vi "add ch config.vi"(7 "range":string[](array[string]), 8 "CAl":T4, 9 "device chanel":T5 {"display" format="%b"}, 10 "value":string[](array[string]), 11 "Enum":T6=enum."CName") -> (2 "device chanel out":T5 {"display" format="%b"})   [LabVIEW 2011]
uses:
  singlechtype.ctl
  config table enum.ctl
  signal type.ctl
  gain.ctl
panel:
  in  "Enum 2":T1(ring)=enum."><（在范围外）"
  in  "Gain":T2
  in  "type":T3
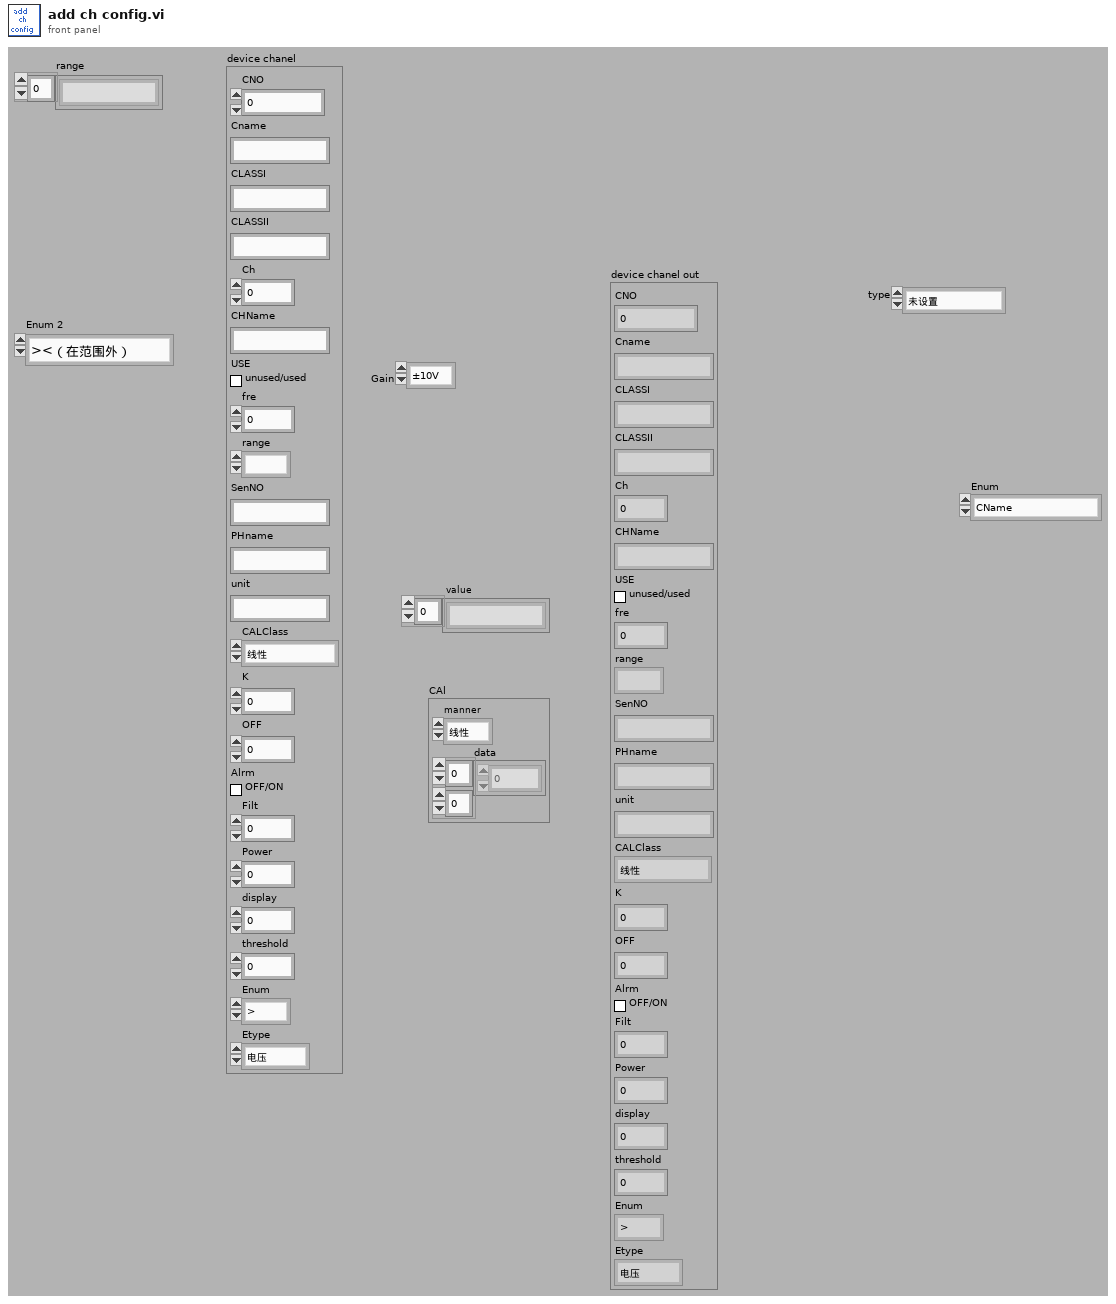
[diagram p1: front panel]
types:
  T1 = enum16{">", ">=", "<", "<=", "<>(在范围内）", "><（在范围外）"}
  T2 = typedef "gain.ctl" = enum16{"±10V", "±5V", "±2.5V", "±1V", "±500mV", "±100mV", "10V", "5V", "2.5V", "1V", "500mV", "100mV"}
  T3 = typedef "signal type.ctl" = enum16{"未设置", "volet", "current", "vibration", "electric charge ", "resistance "}
  T4 = cluster{"manner":enum16{"线性", "查表"}, "data":dbl[][]}
  T5 = typedef "singlechtype.ctl" = cluster{"CNO":u8, "Cname":string, "CLASSI":string, "CLASSII":string, "Ch":u8, "CHName":string, "USE":bool, "fre":dbl, "range":enum16{""}, "SenNO":string, "PHname":string, "unit":string, "CALClass":enum8{"线性", "查表", "公式"}, "K":dbl, "OFF":dbl, "Alrm":bool, "Filt":dbl, "Power":u8, "display":u8, "threshold ":dbl, "Enum":enum16{">", ">=", "<", "<=", "<>(在范围内）", "><（在范围外）"}, "Etype":enum16{"电压", "电流", "电阻", "热电偶K", "热电偶T"}}
  T6 = typedef "config table enum.ctl" = enum16{"CNO.", "CName", "CLASSI", "CLASSII", "ch", "Chname", "USE", "fre", "range", "senNO", "PHname", "unit", "CALclass", "K", "OFF", "Alrm", "filt", "Power", "display", "threshold", "compare", "Etype"}
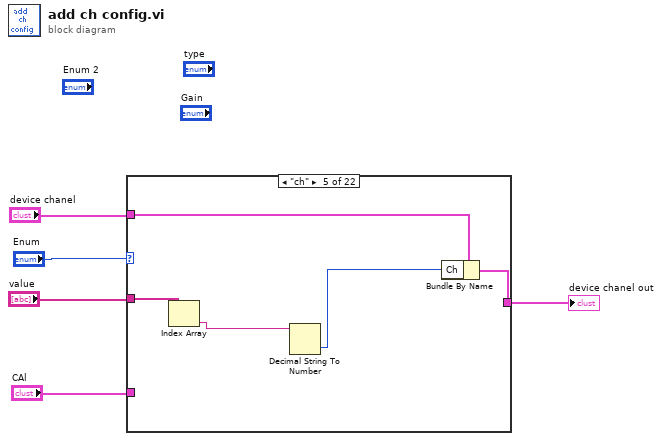
[diagram p0: block diagram]
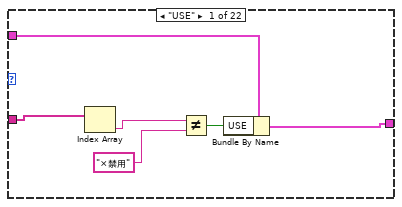
[diagram p2: hidden frame]
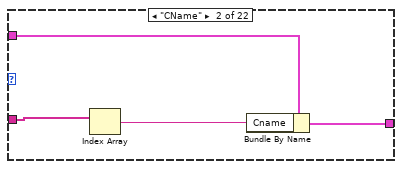
[diagram p3: hidden frame]
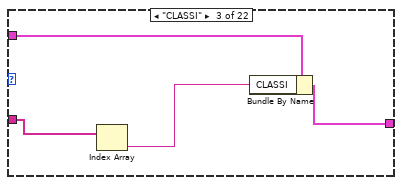
[diagram p4: hidden frame]
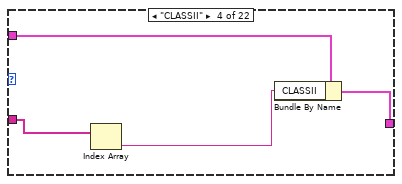
[diagram p5: hidden frame]
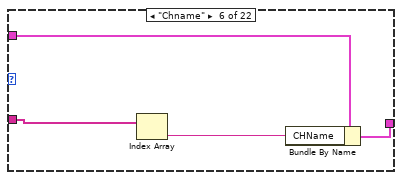
[diagram p6: hidden frame]
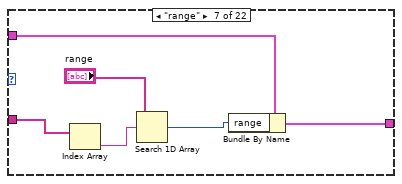
[diagram p7: hidden frame]
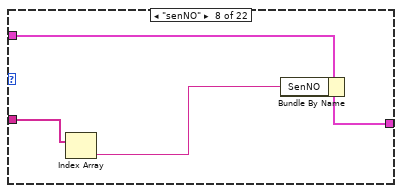
[diagram p8: hidden frame]
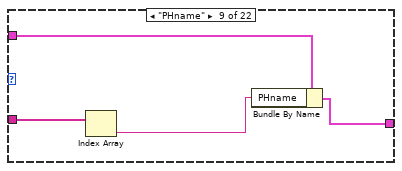
[diagram p9: hidden frame]
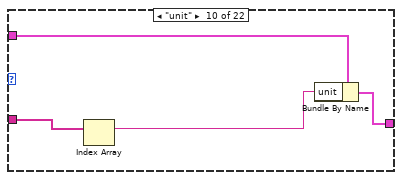
[diagram p10: hidden frame]
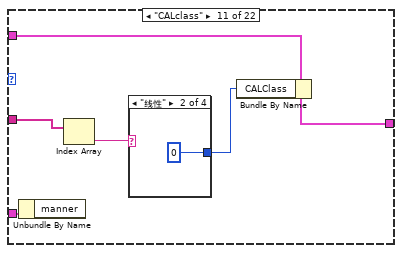
[diagram p11: hidden frame]
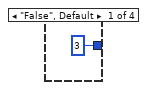
[diagram p12: hidden frame]
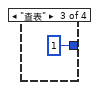
[diagram p13: hidden frame]
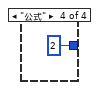
[diagram p14: hidden frame]
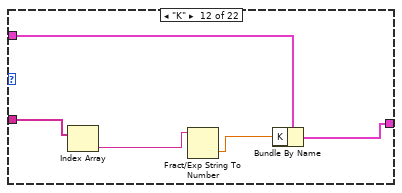
[diagram p15: hidden frame]
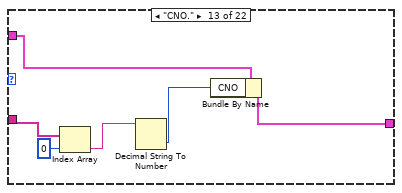
[diagram p16: hidden frame]
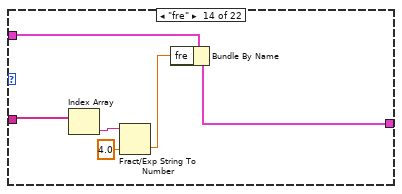
[diagram p17: hidden frame]
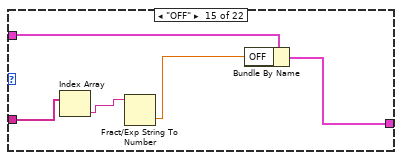
[diagram p18: hidden frame]
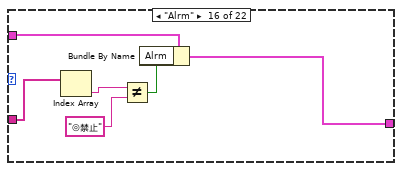
[diagram p19: hidden frame]
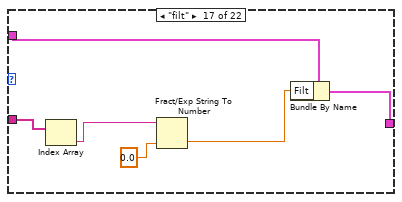
[diagram p20: hidden frame]
diagram:
  n1 = case shown="\"ch\"" "Enum" {
    tunnel: "device chanel" -> [w11 w14 w19 w23 w28 w32 w38 w41 w46 w49 w54 w64 w70 w77 w82 w88 w94 w98 w103 w111 w116 w124]
    tunnel: [w10 w15 w18 w22 w27 w31 w37 w42 w45 w50 w53 w63 w71 w76 w81 w87 w93 w99 w102 w112 w117 w123] -> w2
    tunnel: "value" -> [w6 w13 w16 w21 w26 w29 w36 w40 w44 w48 w56 w65 w69 w75 w78 w83 w92 w100 w108 w113 w119 w122]
    tunnel: "CAl" -> [_ _ _ _ _ _ _ _ _ _ w55 _ _ _ _ _ _ _ _ _ _ _]
    frame "USE" {
      n2 = Index Array(array=w6) -> (element=w9:string)  [unwired: 1 in]
      n3 = Not Equal?(x=w9, y="×禁用") -> (x != y?=w8:bool)
      n4 = Bundle By Name(cluster=w11, "USE"=w8) -> (w10:T5)
    }
    frame "CName" {
      n5 = Index Array(array=w13) -> (element=w12:string)  [unwired: 1 in]
      n6 = Bundle By Name(cluster=w14, "Cname"=w12) -> (w15:T5)
    }
    frame "CLASSI" {
      n7 = Index Array(array=w16) -> (element=w17:string)  [unwired: 1 in]
      n8 = Bundle By Name(cluster=w19, "CLASSI"=w17) -> (w18:T5)
    }
    frame "CLASSII" {
      n9 = Index Array(array=w21) -> (element=w20:string)  [unwired: 1 in]
      n10 = Bundle By Name(cluster=w23, "CLASSII"=w20) -> (w22:T5)
    }
    frame "ch" {
      n11 = Index Array(array=w26) -> (element=w25:string)  [unwired: 1 in]
      n12 = Decimal String To Number(string=w25) -> (number=w24:i32)  [unwired: 2 in, 1 out]
      n13 = Bundle By Name(cluster=w28, "Ch"=w24) -> (w27:T5)
    }
    frame "Chname" {
      n14 = Index Array(array=w29) -> (element=w30:string)  [unwired: 1 in]
      n15 = Bundle By Name(cluster=w32, "CHName"=w30) -> (w31:T5)
    }
    frame "range" {
      n16 = Index Array(array=w36) -> (element=w35:string)  [unwired: 1 in]
      n17 = Search 1D Array(1D array="range", element=w35) -> (index of element=w34:i32)  [unwired: 1 out]
      n18 = Bundle By Name(cluster=w38, "range"=w34) -> (w37:T5)
    }
    frame "senNO" {
      n19 = Index Array(array=w40) -> (element=w39:string)  [unwired: 1 in]
      n20 = Bundle By Name(cluster=w41, "SenNO"=w39) -> (w42:T5)
    }
    frame "PHname" {
      n21 = Index Array(array=w44) -> (element=w43:string)  [unwired: 1 in]
      n22 = Bundle By Name(cluster=w46, "PHname"=w43) -> (w45:T5)
    }
    frame "unit" {
      n23 = Index Array(array=w48) -> (element=w47:string)  [unwired: 1 in]
      n24 = Bundle By Name(cluster=w49, "unit"=w47) -> (w50:T5)
    }
    frame "CALclass" {
      n25 = Unbundle By Name(w55) -> ()  [unwired: 1 out]
      n26 = Index Array(array=w56) -> (element=w52:string)  [unwired: 1 in]
      n27 = case shown="\"线性\"" w52 {
        tunnel: [3 0 1 2] -> w51
        frame "False", Default {
        }
        frame "线性" {
        }
        frame "查表" {
        }
        frame "公式" {
        }
      }
      n28 = Bundle By Name(cluster=w54, "CALClass"=w51) -> (w53:T5)
    }
    frame "K" {
      n29 = Index Array(array=w65) -> (element=w61:string)  [unwired: 1 in]
      n30 = Fract/Exp String To Number(string=w61) -> (number=w62:dbl)  [unwired: 3 in, 1 out]
      n31 = Bundle By Name(cluster=w64, "K"=w62) -> (w63:T5)
    }
    frame "CNO." {
      n32 = Index Array(array=w69, index=0) -> (element=w68:string)
      n33 = Decimal String To Number(string=w68) -> (number=w67:i32)  [unwired: 2 in, 1 out]
      n34 = Bundle By Name(cluster=w70, "CNO"=w67) -> (w71:T5)
    }
    frame "fre" {
      n35 = Index Array(array=w75) -> (element=w74:string)  [unwired: 1 in]
      n36 = Fract/Exp String To Number(string=w74, default (0 dbl)=4.0 ("default (0 DBL)")) -> (number=w73:dbl)  [unwired: 3 out]
      n37 = Bundle By Name(cluster=w77, "fre"=w73) -> (w76:T5)
    }
    frame "OFF" {
      n38 = Index Array(array=w78) -> (element=w80:string)  [unwired: 1 in]
      n39 = Fract/Exp String To Number(string=w80) -> (number=w79:dbl)  [unwired: 4 out]
      n40 = Bundle By Name(cluster=w82, "OFF"=w79) -> (w81:T5)
    }
    frame "Alrm" {
      n41 = Index Array(array=w83) -> (element=w86:string)  [unwired: 1 in]
      n42 = Not Equal?(x=w86, y="◎禁止") -> (x != y?=w84:bool)
      n43 = Bundle By Name(cluster=w88, "Alrm"=w84) -> (w87:T5)
    }
    frame "filt" {
      n44 = Index Array(array=w92) -> (element=w91:string)  [unwired: 1 in]
      n45 = Fract/Exp String To Number(string=w91, default (0 dbl)=0.0 ("default (0 DBL)")) -> (number=w90:dbl)  [unwired: 2 in, 1 out]
      n46 = Bundle By Name(cluster=w94, "Filt"=w90) -> (w93:T5)
    }
    frame "Power" {
      n47 = Index Array(array=w100) -> (element=w97:string)  [unwired: 1 in]
      n48 = Decimal String To Number(string=w97, default (0L)=0 ("default (0 I32)")) -> (number=w96:i32)  [unwired: 1 in, 1 out]
      n49 = Bundle By Name(cluster=w98, "Power"=w96) -> (w99:T5)
    }
    frame "display" {
      n50 = Array Subset(array=w108, length=8) -> (w106:string[])  [unwired: 1 in]
      n51 = Equal?(x=w106, y="是") -> (x = y?=w104:bool[])
      n52 = Boolean Array To Number(Boolean array=w104) -> (number=w101:u32)
      n53 = Bundle By Name(cluster=w103, "display"=w101) -> (w102:T5)
    }
    frame "threshold" {
      n54 = Index Array(array=w113) -> (element=w110:string)  [unwired: 1 in]
      n55 = Fract/Exp String To Number(string=w110) -> (number=w109:dbl)  [unwired: 3 in, 1 out]
      n56 = Bundle By Name(cluster=w111, "threshold"=w109) -> (w112:T5)
    }
    frame "compare" {
      n57 = property on="Enum 2" class="Enum (strict)"() -> ("Strings []"=w114:string[])  [unwired: 2 in, 2 out]
      n58 = Index Array(array=w119) -> (element=w118:string)  [unwired: 1 in]
      n59 = Search 1D Array(1D array=w114, element=w118) -> (index of element=w115:i32)  [unwired: 1 in]
      n60 = Bundle By Name(cluster=w116, "Enum"=w115) -> (w117:T5)
    }
    frame "Etype", Default {
      n61 = Index Array(array=w122) -> (element=w121:string)  [unwired: 1 in]
      n62 = Decimal String To Number(string=w121) -> (number=w120:i32)  [unwired: 2 in, 1 out]
      n63 = Bundle By Name(cluster=w124, "Etype"=w120) -> (w123:T5)
    }
  }
  "device chanel out" <- w2
